vi "headers.vi"(8 "error in":errorcluster, 9 "Number of Columns":i32, 10 "Column Headers":string[](array[string]), 11 "AppendTable":refnum<k7>) -> (0 "error out":errorcluster)   [LabVIEW 2017, in "NI_ReportGenerationCore.lvlib"]
uses:
  <vilib>/Utility/NIReport.llb/NI_ReportGenerationCore.lvlib
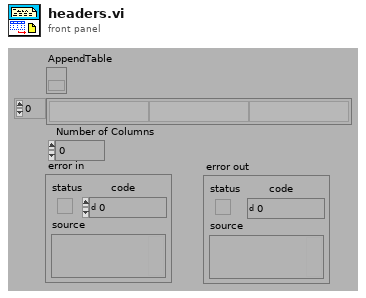
[diagram p1: front panel]
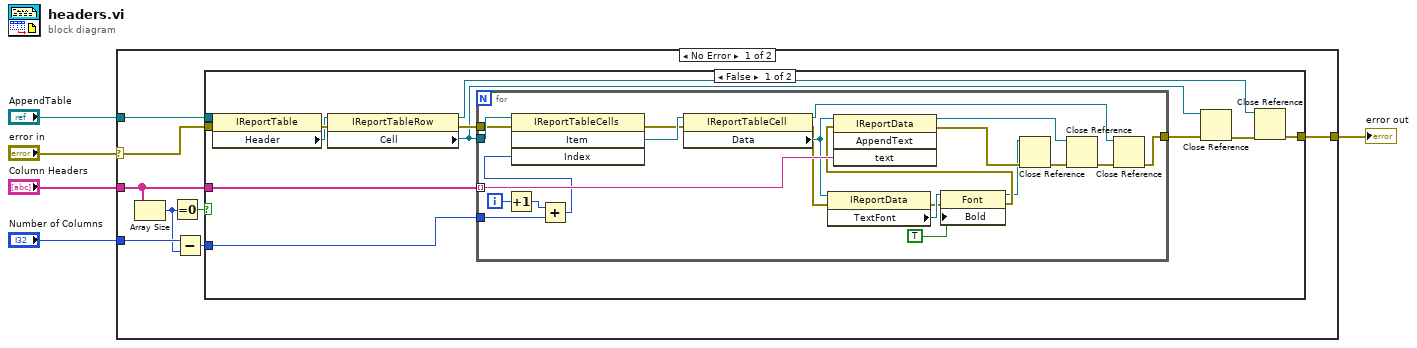
[diagram p0: block diagram]
diagram:
  n1 = case shown="No Error" "error in" {
    selector: "error in" -> [w6 w49]
    tunnel: "AppendTable" -> [w13 _]
    tunnel: [w12 w49] -> w4
    tunnel: "Column Headers" -> [w10 _]
    tunnel: "Number of Columns" -> [w8 _]
    frame No Error {
      n2 = Array Size(array=w10) -> (size(s)=w7:i32)
      n3 = Equal To 0?(x=w7) -> (x = 0?=w11:bool)
      n4 = Subtract(x=w8, y=w7) -> (x-y=w9:i32)
      n5 = case shown="False" w11 {
        tunnel: w6 -> [w25 w48]
        tunnel: w13 -> [w22 _]
        tunnel: w10 -> [w21 _]
        tunnel: [w17 w48] -> w12
        tunnel: w9 -> [w19 _]
        frame False {
          n6 = property class="IReportTable"(reference=w22, error in=w25) -> (error out=w24:errorcluster, "Header"=w23:refnum<k7>)  [unwired: 1 out]
          n7 = property class="IReportTableRow"(reference=w23, error in=w24) -> (reference out=w18:refnum<k7>, error out=w20:errorcluster, "Cell"=w14:refnum<k7>)
          n8 = for {
            tunnel: w14 -> [w45]
            tunnel: w21 -> [w42] mode=indexing
            tunnel: w20 -> [w44]
            tunnel: [w26] -> w16
            tunnel: w19 -> [w35]
            i -> [w47]
            n9 = Increment(x=w47) -> (x+1=w34:i32)
            n10 = Add(x=w34, y=w35) -> (x+y=w33:i32)
            n11 = invoke class="IReportTableCells" method="Item"(reference=w45, error in=w44, "Index"=w33) -> (error out=w43:errorcluster, "Item"=w46:refnum<k7>)  [unwired: 1 in, 2 out]
            n12 = property class="IReportTableCell"(reference=w46, error in=w43) -> (reference out=w30:refnum<k7>, error out=w37:errorcluster, "Data"=w41:refnum<k7>)
            n13 = property class="IReportData"(reference=w41, error in=w37) -> (error out=w38:errorcluster, "TextFont"=w40:refnum<k7>)  [unwired: 1 out]
            n14 = property class="Font"(reference=w40, error in=w38, "Bold"=TRUE) -> (reference out=w27:refnum<k7>, error out=w36:errorcluster)
            n15 = invoke class="IReportData" method="AppendText"(reference=w41, error in=w36, "text"=w42) -> (reference out=w31:refnum<k7>, error out=w29:errorcluster)  [unwired: 1 in, 2 out]
            n16 = Close Reference(reference=w27, error in (no error)=w29) -> (error out=w28:errorcluster)
            n17 = Close Reference(reference=w31, error in (no error)=w28) -> (error out=w32:errorcluster)
            n18 = Close Reference(reference=w30, error in (no error)=w32) -> (error out=w26:errorcluster)
          }
          n19 = Close Reference(reference=w14, error in (no error)=w16) -> (error out=w15:errorcluster)
          n20 = Close Reference(reference=w18, error in (no error)=w15) -> (error out=w17:errorcluster)
        }
        frame True {
        }
      }
    }
    frame Error {
    }
  }
  "error out" <- w4
